vi "isLeapYear.vi"(11 "year":string) -> (3 "Boolean":bool)   [LabVIEW 2013, in "UI_TimeSelector.xctl"]
uses:
  UI_TimeSelector.xctl
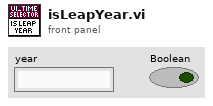
[diagram p1: front panel]
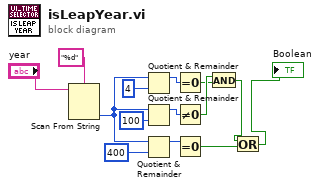
[diagram p0: block diagram]
diagram:
  n1 = Scan From String(format string="%d", input string="year") -> (output 1=w3:i32)  [unwired: 3 in, 3 out]
  n2 = Quotient & Remainder(x=w3, y=4) -> (x-y*floor(x/y)=w7:i32)  [unwired: 1 out]
  n3 = Quotient & Remainder(x=w3, y=100) -> (x-y*floor(x/y)=w9:i32)  [unwired: 1 out]
  n4 = Quotient & Remainder(x=w3, y=400) -> (x-y*floor(x/y)=w8:i32)  [unwired: 1 out]
  n5 = Equal To 0?(x=w7) -> (x = 0?=w10:bool)
  n6 = Not Equal To 0?(x=w9) -> (x != 0?=w11:bool)
  n7 = Equal To 0?(x=w8) -> (x = 0?=w13:bool)
  n8 = And(x=w11, y=w10) -> (x .and. y?=w12:bool)
  n9 = Or(x=w12, y=w13) -> (x .or. y?=→"Boolean":bool)
